vi "Tosca-Stop.vi"(11 "error in (no error)":errorcluster) -> (15 "error out":errorcluster)   [LabVIEW 2020]
uses:
  epl-vi-lib/PXI DAQ VIs/AODO/Typedefs/AODO-Action.ctl
  PXI DAQ VIs/TDT VIs/TDT AODO VIs/Typedefs/TDT-AODO-Action.ctl
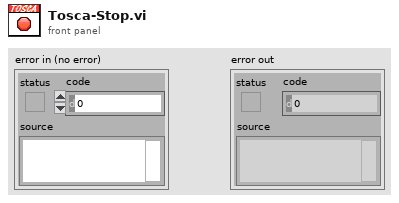
[diagram p1: front panel]
types:
  T1 = typedef "TDT-AODO-Action.ctl" = enum16{"Configure", "Initialize", "Start", "Stop", "Write", "Clean up", "Space available"}
  T2 = typedef "AODO-Action.ctl" = enum16{"Configure", "Initialize", "Start", "Write", "Clean up", "Init & Start", "Config & Test", "Position", "Set AO Gains", "Zero", "Prime", "Status"}
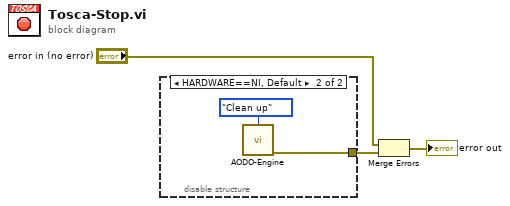
[diagram p0: block diagram]
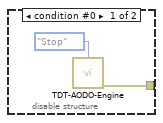
[diagram p2: hidden frame]
diagram:
  n1 = disable-structure shown="HARDWARE==NI, Default" {
    disable-tunnel: [w5 w6] -> w3
    frame condition #0 {
      n2 = call "TDT-AODO-Engine.vi"("Action"=TDT-AODO-Action."Stop") -> ("error out"=w5:errorcluster)  [unwired: 12 in, 2 out]
    }
    frame condition #1 (active) {
      n3 = call "AODO-Engine.vi"("Action"=AODO-Action."Clean up") -> ("error out"=w6:errorcluster)  [unwired: 10 in, 4 out]
    }
  }
  n4 = Merge Errors("error in (no error)", w3) -> (→"error out":errorcluster)
